vi "Convert to Waveform Function Test.vi"() -> ()   [LabVIEW 2020]
panel:
  out "Waveform Graph":waveform(dbl)[](graph)
  out "Array":waveform(dbl)[](array[waveform])
  in  "stop":bool
  out "Data":dbl[][](array[numeric]) format="%.3f"
  out "Error Message":string
  out "Stream Parameters":T1 {"Device Backlog [%]" format="%.2f"}
  out "Actual Scan Rate (Hz)":dbl=1000.0 format="%.3f"
  in  "Scan Rate (Hz)":dbl=1000.0 format="%.3f"
  in  "Display Rate (Hz)":i32=1
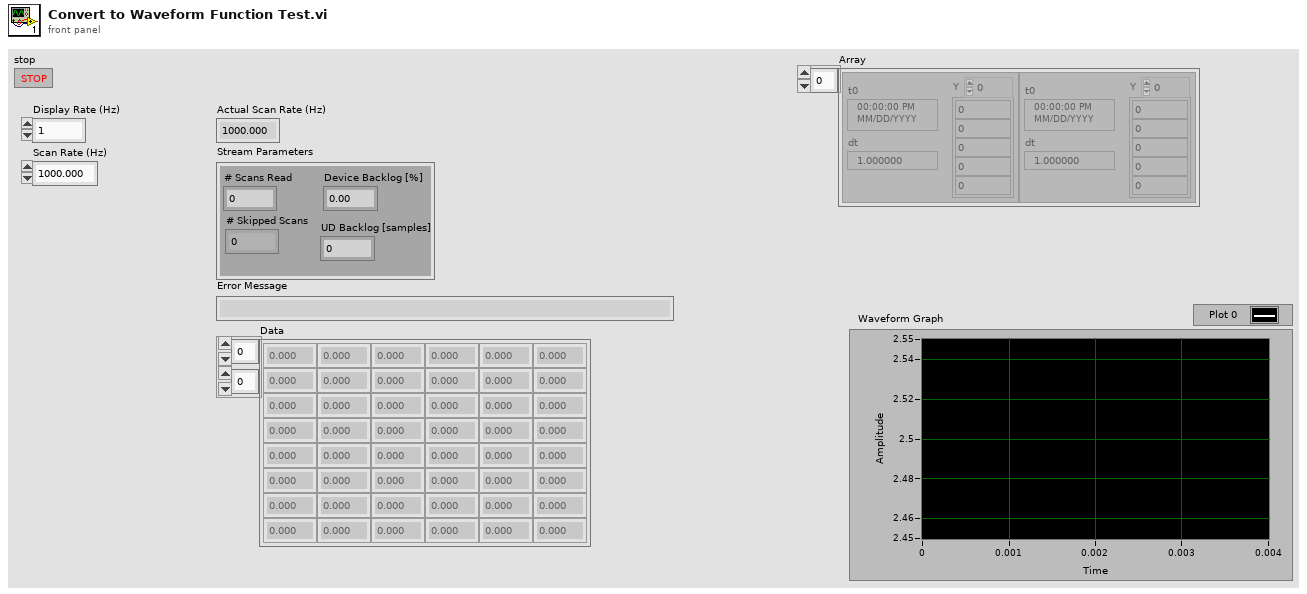
[diagram p1: front panel]
types:
  T1 = cluster{"# Scans Read":i32, "# Skipped Scans":i32, "Device Backlog [%]":dbl, "UD Backlog [samples]":i32}
  T2 = cluster{"DeviceType":i32, "Connection Type":u16, "Address":string, "FirstFound":bool}
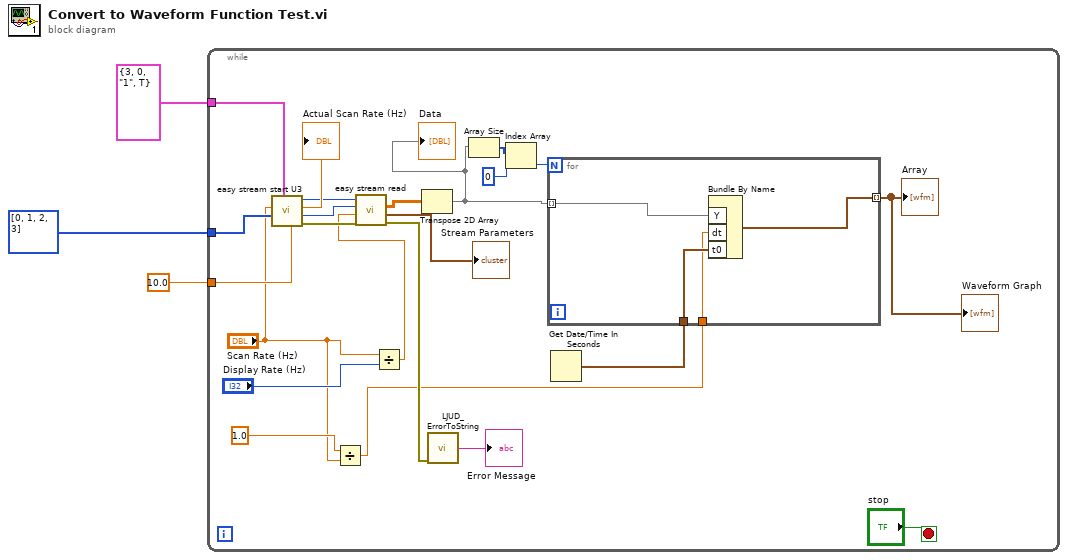
[diagram p0: block diagram]
diagram:
  n1 = while {
    tunnel: T2 {"DeviceType"=3, "Connection Type"=0, "Address"="1", "FirstFound"=TRUE} ("Device Info") -> [w23]
    tunnel: 10.0 ("PC buffer size (seconds)") -> [w22]
    tunnel: u8[] [0, 1, 2, 3] ("Scan List (+)") -> [w14]
    stop <- "stop" stop-if-true
    n2 = call "easy stream start U3.vi"("PC buffer size (seconds)"=w22, "Device Info"=w23, "Scan List (+)"=w14, "Scan Rate (Hz)"="Scan Rate (Hz)") -> ("error out"=w25:errorcluster, "# Channels"=w21:i32, "Actual Scan Rate (Hz)"=→"Actual Scan Rate (Hz)":dbl, "Handle Out"=w24:i32)  [unwired: 4 in]
    n3 = Divide(x=1.0, y="Scan Rate (Hz)") -> (x/y=w5:dbl)
    n4 = Divide(x="Scan Rate (Hz)", y="Display Rate (Hz)") -> (x/y=w8:dbl)
    n5 = call "easy stream read.vi"("error in"=w25, "Scans To Read"=w8, "# Channels In Stream"=w21, "Handle In"=w24) -> ("error out"=w20:errorcluster, "Stream Parameters"=→"Stream Parameters":T1, "Data"=w11:dbl[][])  [unwired: 4 in, 1 out]
    n6 = Transpose 2D Array(2D array=w11) -> (transposed array=w10:dbl[][])
    "Data" <- w10
    n7 = call "LJUD_ErrorToString.vi"("error in"=w20) -> ("String"=→"Error Message":string)  [unwired: 10 in]
    n8 = Array Size(array=w10) -> (size(s)=w17:i32[])
    n9 = Index Array(array=w17, index=0) -> (element=w16:i32)
    n10 = Get Date/Time In Seconds() -> (seconds since 1Jan1904=w15:timestamp)
    n11 = for {
      N: w16 -> [_]
      tunnel: w10 -> [w30] mode=indexing
      tunnel: [w27] -> w4 mode=indexing
      tunnel: w15 -> [w29]
      tunnel: w5 -> [w28]
      n12 = Bundle By Name("Y"=w30, "dt"=w28, "t0"=w29) -> (w27:waveform(dbl))  [unwired: 1 in]
    }
    "Array" <- w4
    "Waveform Graph" <- w4
  }
